vi "AR Drone - Simple NavData.vi"() -> ()   [LabVIEW 2014]
doc: "Very simple example showing how to use the base VIs to control the AR Drone and receive and display navigation data."
uses:
  <vilib>/LVH/AR Drone Toolkit/Decode NavData/Typedefs/NavData Demo.ctl
  <vilib>/LVH/AR Drone Toolkit/AR Drone.lvlib
panel:
  out "Unf. vx":sgl(graph)
  out "Unf. vy":sgl(graph)
  out "Velocity y":dynamicdata(graph)
  out "Altitude":u32(graph)
  out "Velocity x":dynamicdata(graph)
  in  "Setup Parameters":T1={"Drone IP address"="192.168.1.1", "Home IP address"="192.168.1.2", "Flight Mode"=enum."INDOOR MODE", "Mounted Hull"=enum."INDOOR HULL", "Video Camera"=1, "Max Altitude (m)"=3.0, "Max Pitch and Roll Angle (deg)"=10.0, "Max Vertical Speed (m/s)"=0.7, "Max Yaw Speed (deg/s)"=100.0} {"Video Camera" items=["Bottom Camera"=1, "Front Camera"=0, "Front in Bottom"=3, "Bottom in Front"=2]}
  out "Tilt":T2(graph)
  in  "device ID":i32=3
  out "Battery Remaining":dbl(slide) scale=0.0..100.0
  out "NavData Out":T3
  in  "stop":bool
  in  "Emergency Landing":bool
  in  "Take Off/Land":bool
  in  "Hover":bool
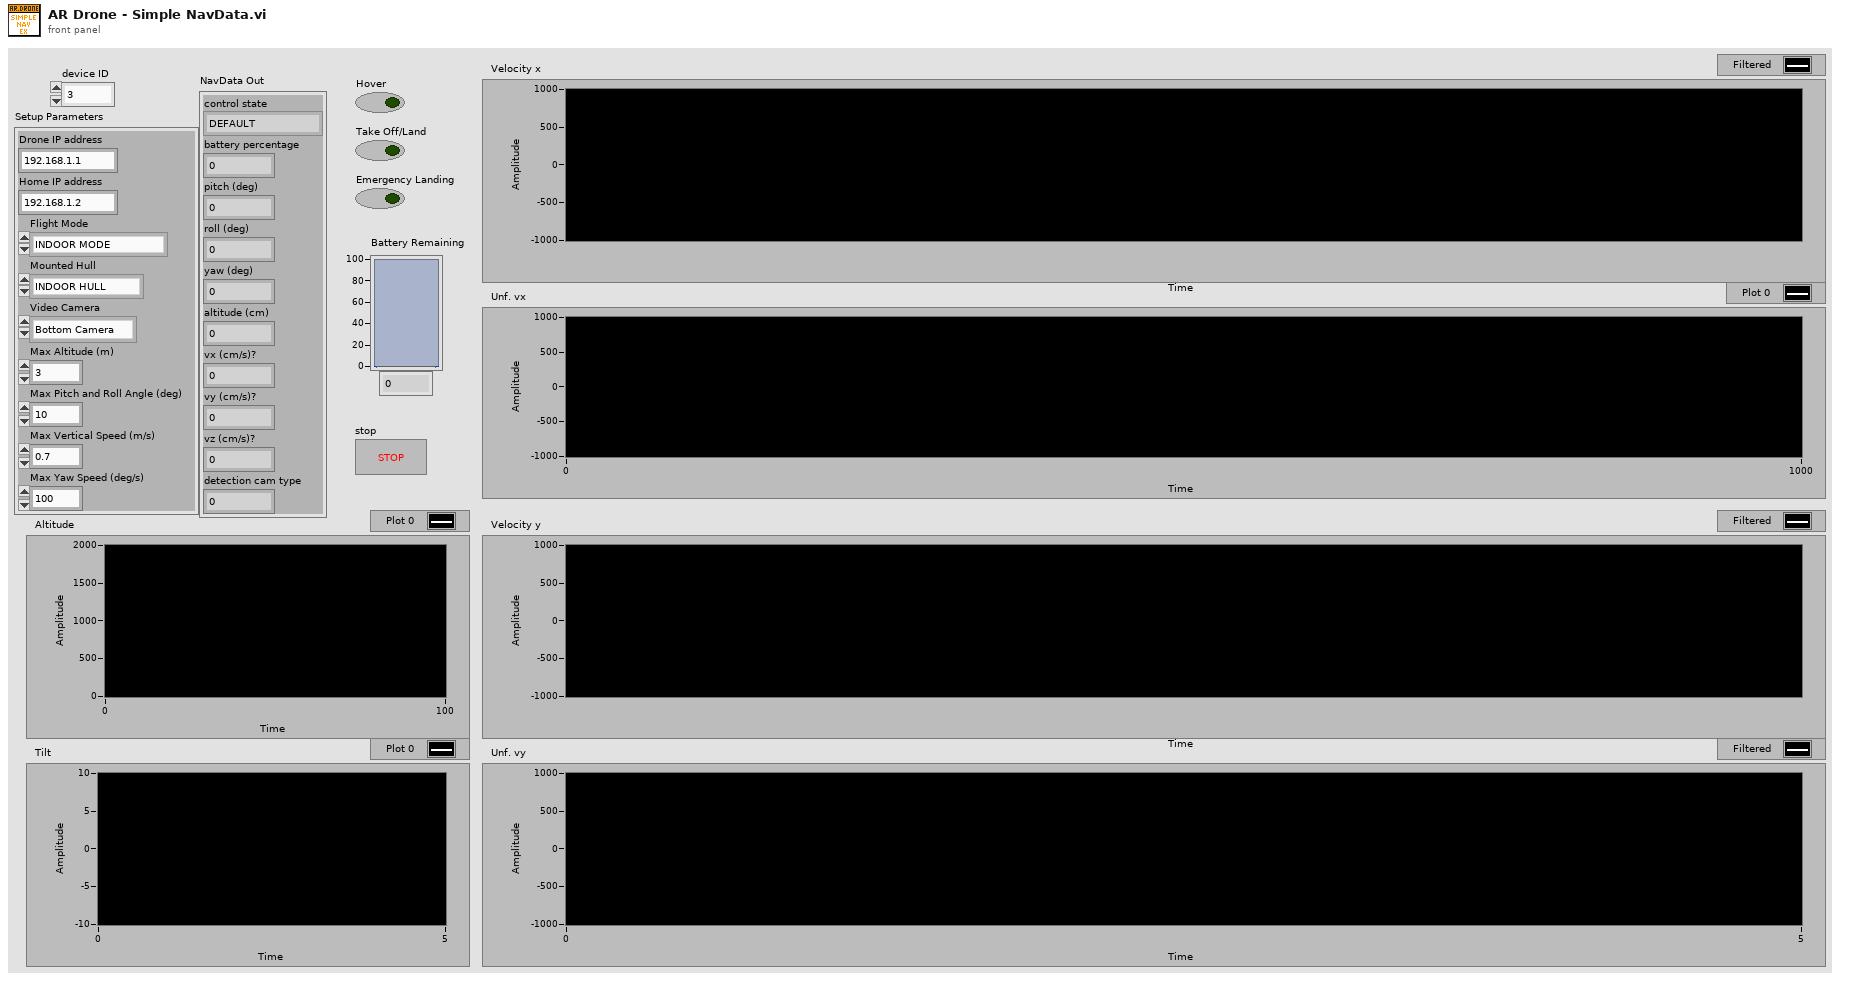
[diagram p1: front panel]
types:
  T1 = cluster{"Drone IP address":string, "Home IP address":string, "Flight Mode":enum8{"OUTDOOR MODE", "INDOOR MODE"}, "Mounted Hull":enum8{"OUTDOOR HULL", "INDOOR HULL"}, "Video Camera":u8, "Max Altitude (m)":sgl, "Max Pitch and Roll Angle (deg)":sgl, "Max Vertical Speed (m/s)":sgl, "Max Yaw Speed (deg/s)":sgl}
  T2 = cluster{"pitch (deg)":sgl, "roll (deg)":sgl, "yaw (deg)":sgl}
  T3 = typedef "AR Drone.lvlib/NavData Demo.ctl" = cluster{"control state":enum32{"DEFAULT", "INIT", "LANDING", "FLYING", "HOVERING", "TEST", "TRANS_TAKEOFF", "TRANS_GOTOFIX", "TRANS_LANDING"}, "battery percentage":u32, "pitch (deg)":sgl, "roll (deg)":sgl, "yaw (deg)":sgl, "altitude (cm)":u32, "vx (cm/s)?":sgl, "vy (cm/s)?":sgl, "vz (cm/s)?":sgl, "detection cam type":u32}
  T4 = typedef "AR Drone.lvlib/AR Drone Resource.ctl" = cluster{"UDP Control Connection":refnum<k16>, "UDP NavData Connection":refnum<k16>, "UDP Video Connection (Drone 1.0)":refnum<k16>, "TCP Video Connection (Drone 2.0)":refnum<k5>, "TCP Control Port Connection":refnum<k5>, "Drone IP address":string, "Drone Command Port":u16, "Drone NavData Port":u16, "Drone Vid Stream Port":u16, "Drone TCP Control Port":u16, "Home IP address":string, "Home Command Port":u16, "Home NavData Port":u16, "Home Vid Stream Port":u16, "Drone Version":i32, "Drone Index":i32, "Command Sequence":i32}
  T5 = cluster{"Roll":dbl, "Pitch":dbl, "Vertical Speed":dbl, "Yaw Speed":dbl}
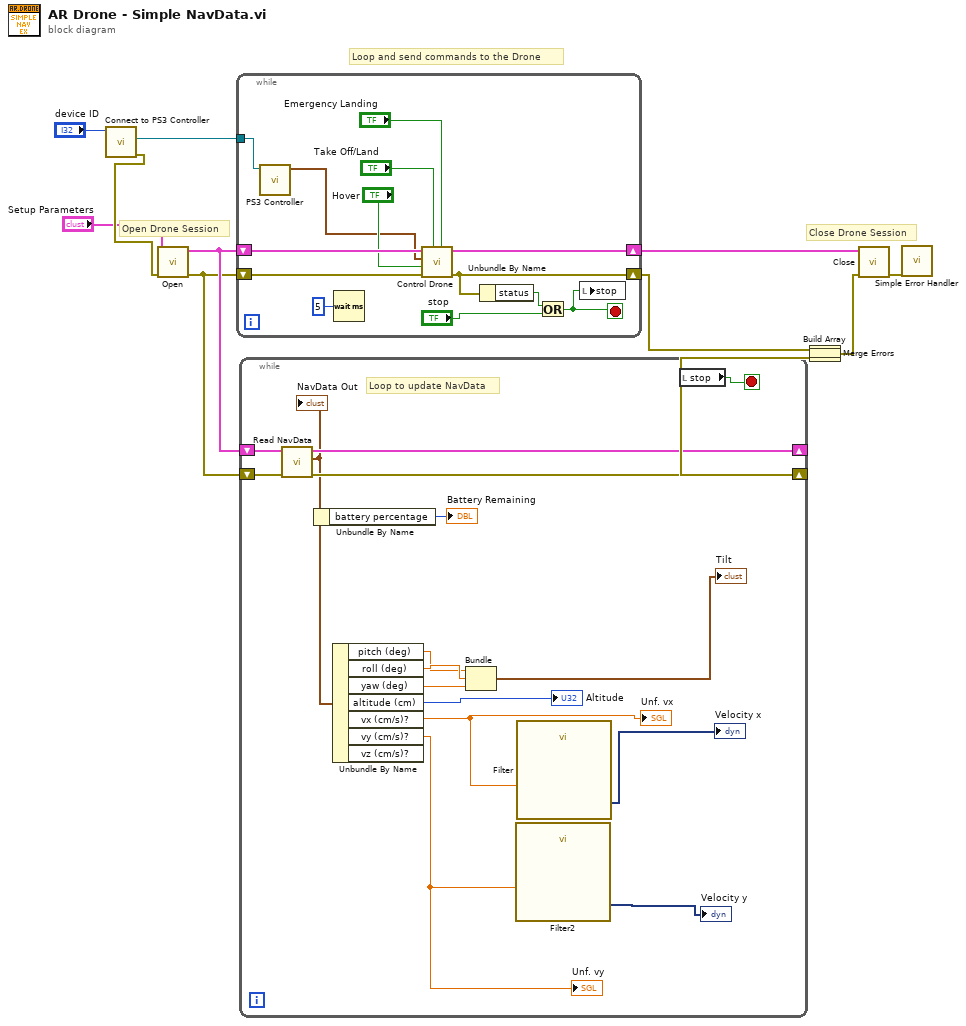
[diagram p0: block diagram]
diagram:
  # "Close Drone Session"
  # "Loop and send commands to the Drone"
  # "Open Drone Session"
  n1 = call "Connect to PS3 Controller.vi"("device ID"="device ID") -> ("error out"=w2:errorcluster, "device ID 2"=w4:refnum<k1>)  [unwired: 7 in, 1 out]
  n2 = call <vilib>:"Open.vi"("error in (no error)"=w2, "Setup Parameters"="Setup Parameters") -> ("error out"=w10:errorcluster, "AR Drone Resource"=w11:T4)  [unwired: 8 in]
  n3 = while {
    shift-right: [w20] -> w12
    shift-left: w11 -> [w24]
    shift-right: [w16] -> w8
    shift-left: w10 -> [w25]
    tunnel: w4 -> [w13]
    stop <- w15 stop-if-true
    n4 = call "PS3 Controller.vi"("device ID"=w13) -> ("Control cluster"=w14:T5)  [unwired: 7 in, 3 out]
    n5 = Wait (ms)(milliseconds to wait=u32 5) -> ()  [unwired: 1 out]
    n6 = call <vilib>:"Control Drone.vi"("Emergency Landing"="Emergency Landing", "Takeoff/Land"="Take Off/Land", "error in (no error)"=w25, "Hover"="Hover", "Control Cluster"=w14, "AR Drone Resource"=w24) -> ("error out"=w16:errorcluster, "AR Drone Resource Out"=w20:T4)  [unwired: 4 in]
    n7 = Unbundle By Name(w16) -> ("status"=w18:bool)
    n8 = Or(x=w18, y="stop") -> (x .or. y?=w15:bool)
    n9 = local write "stop"(w15) -> ()
  }
  n10 = while {
    shift-right: [w39] -> _
    shift-left: w11 -> [w40]
    shift-right: [w37] -> w9
    shift-left: w10 -> [w38]
    stop <- w41 stop-if-true
    # "Loop to update NavData"
    n11 = call <vilib>:"Read NavData.vi"("error in (no error)"=w38, "AR Drone Resource"=w40) -> ("error out"=w37:errorcluster, "NavData Out"=w35:T3, "AR Drone Resource Out"=w39:T4)  [unwired: 7 in]
    "NavData Out" <- w35
    n12 = Unbundle By Name(w35) -> ("battery percentage"=→"Battery Remaining":u32)
    n13 = Unbundle By Name(w35) -> ("pitch (deg)"=w31:sgl, "roll (deg)"=w34:sgl, "yaw (deg)"=w33:sgl, "altitude (cm)"=→"Altitude":u32, "vx (cm/s)?"=w26:sgl, "vy (cm/s)?"=w27:sgl)  [unwired: 1 out]
    "Unf. vy" <- w27
    "Unf. vx" <- w26
    n14 = Bundle("pitch (deg)"=w31, "roll (deg)"=w34, "yaw (deg)"=w33) -> (→"Tilt":T2)  [unwired: 1 in]
    n15 = call "Filter2"("Signal"=w27) -> ("Filtered Signal"=→"Velocity y":dynamicdata)  [unwired: 9 in, 1 out]
    n16 = call "Filter"("Signal"=w26) -> ("Filtered Signal"=→"Velocity x":dynamicdata)  [unwired: 9 in, 1 out]
    n17 = local read "stop"() -> (w41:bool)
  }
  n18 = Build Array(w8, w9) -> (w5:errorcluster[])
  n19 = Merge Errors(w5) -> (w7:errorcluster)
  n20 = call <vilib>:"Close.vi"("error in (no error)"=w7, "AR Drone Resource"=w12) -> ("error out"=w6:errorcluster)  [unwired: 9 in]
  n21 = call <vilib>:"Simple Error Handler.vi"("error in (no error)"=w6) -> ()  [unwired: 4 in, 5 out]
